vi "Enable Logging.vi"(8 "error in (no error)":errorcluster, 9 "Enable Logging (T:Enable)":bool=TRUE, 10 "Buffer Name (defbuffer1)":string="defbuffer1", 11 "VISA resource name":refnum<visa-resource-name>) -> (0 "error out":errorcluster, 3 "VISA resource name out":refnum<visa-resource-name>)   [LabVIEW 2017, in "Keithley 2450.lvlib"]
doc: "This determines whether the reading buffer should log informational events."
uses:
  Keithley 2450.lvlib
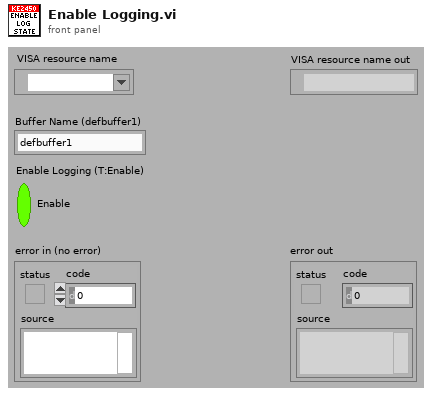
[diagram p1: front panel]
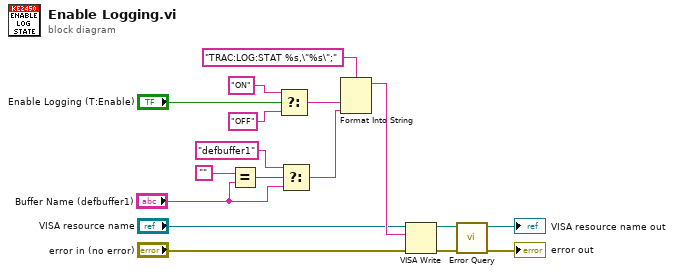
[diagram p0: block diagram]
diagram:
  n1 = Equal?(x="", y="Buffer Name (defbuffer1)") -> (x = y?=w4:bool)
  n2 = Select(t="ON", s="Enable Logging (T:Enable)", f="OFF") -> (s? t:f=w10:string)
  n3 = Select(t="defbuffer1", s=w4, f="Buffer Name (defbuffer1)") -> (s? t:f=w1:string)
  n4 = Format Into String(format string="TRAC:LOG:STAT %s,\"%s\";", w10, w1) -> (resulting string=w9:string)  [unwired: 2 in, 1 out]
  n5 = VISA Write(VISA resource name="VISA resource name", write buffer=w9, error in (no error)="error in (no error)") -> (VISA resource name out=w15:refnum<visa-resource-name>, error out=w14:errorcluster)  [unwired: 1 out]
  n6 = call "Error Query.vi"("error in (no error)"=w14, "VISA resource name"=w15) -> ("error out"=→"error out":errorcluster, "VISA resource name out"=→"VISA resource name out":refnum<visa-resource-name>)  [unwired: 8 out]
